vi "Cut_Zero_Displacement_In_Track_Column-1.vi"(1 "[IN] Track in column":dbl[](array[numeric])) -> (0 "[OUT] Track in column\nwithout zero points":dbl[](array[numeric]))   [LabVIEW 2017]
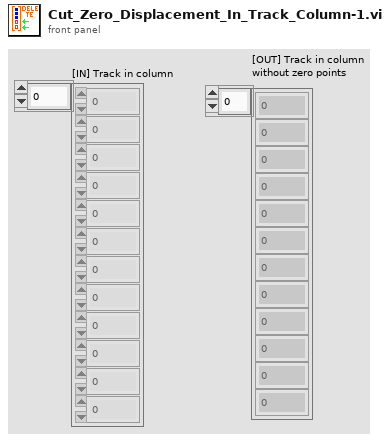
[diagram p1: front panel]
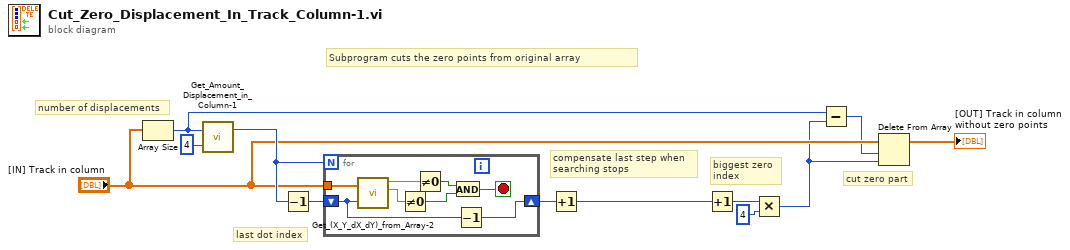
[diagram p0: block diagram]
diagram:
  # "Subprogram cuts the zero points from original array"
  # "cut zero part"
  # "biggest zero \nindex"
  # "compensate last step when \nsearching stops"
  # "last dot index"
  # "number of displacements"
  n1 = Array Size(array="[IN] Track in column") -> (size(s)=w3:i32)
  n2 = call "Get_Amount_Displacement_in_Column-1.vi"("multiplier"=4 ("y"), "# Rows"=w3) -> ("Displ amount"=w9:i32)  [unwired: 1 out]
  n3 = Decrement(x=w9) -> (x-1=w11:i32)
  n4 = for {
    N: w9 -> [_]
    tunnel: "[IN] Track in column" -> [w16]
    shift-right: [w18] -> w10
    shift-left: w11 -> [w13]
    stop <- w17 stop-if-true
    n5 = call "Get_(X_Y_dX_dY)_from_Array-2.vi"("(X,Y,dX,dY)"=w16, "Index of Displacement"=w13) -> ("X"=w15:dbl, "Y"=w14:dbl)  [unwired: 2 out]
    n6 = Not Equal To 0?(x=w14) -> (x != 0?=w19:bool)
    n7 = Not Equal To 0?(x=w15) -> (x != 0?=w20:bool)
    n8 = And(x=w20, y=w19) -> (x .and. y?=w17:bool)
    n9 = Decrement(x=w13) -> (x-1=w18:i32)
  }
  n10 = Increment(x=w10) -> (x+1=w6:i32)
  n11 = Increment(x=w6) -> (x+1=w8:i32)
  n12 = Multiply(x=w8, y=4) -> (x*y=w4:i32)
  n13 = Subtract(x=w3, y=w4) -> (x-y=w2:i32)
  n14 = Delete From Array(array="[IN] Track in column", length=w2, index=w4) -> (array with subset deleted=→"[OUT] Track in column\nwithout zero points":dbl[])  [unwired: 1 out]
